vi "OpenAVIFile.vi"(8 "error in (no error)":errorcluster, 11 "AVI Path":path) -> (0 "error out":errorcluster, 3 "Avi Refnum":T1)   [LabVIEW 2016]
uses:
  <vilib>/vision/Avi1.llb/AviRefnum.ctl
  <vilib>/regexp/Match Regular Expression.xnode
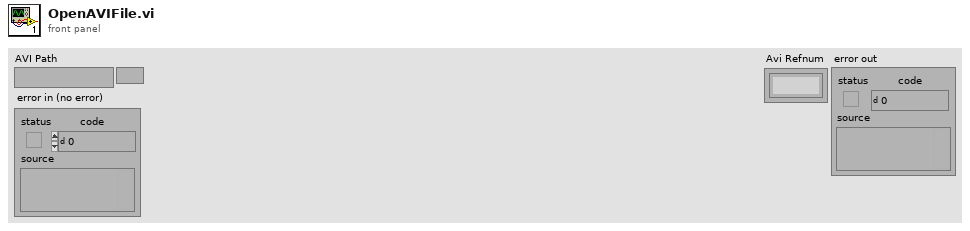
[diagram p1: front panel]
types:
  T1 = typedef "AviRefnum.ctl" = refnum<k1>
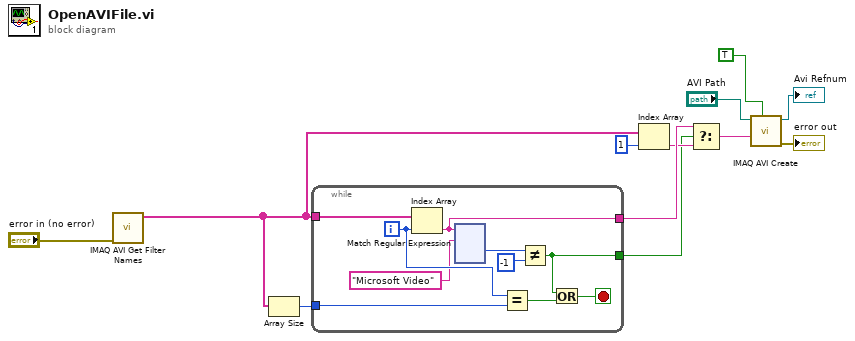
[diagram p0: block diagram]
diagram:
  n1 = call "IMAQ AVI Get Filter Names"("error in (no error)"="error in (no error)") -> ("Filter Names"=w9:string[])  [unwired: 9 in, 1 out]
  n2 = Array Size(array=w9) -> (size(s)=w12:i32)
  n3 = while {
    tunnel: w9 -> [w19]
    tunnel: w12 -> [w22]
    tunnel: [w17] -> w7
    tunnel: [w13] -> w11
    i -> [w18]
    stop <- w21 stop-if-true
    n4 = Index Array(array=w19, index=w18) -> (element=w13:string)
    n5 = xnode "Match Regular Expression"("input string"=w13, "regular expression"="Microsoft Video") -> ("offset past match"=w15:i32)  [unwired: 4 in, 4 out]
    n6 = Equal?(x=w18, y=w22) -> (x = y?=w20:bool)
    n7 = Not Equal?(x=w15, y=-1) -> (x != y?=w17:bool)
    n8 = Or(x=w17, y=w20) -> (x .or. y?=w21:bool)
  }
  n9 = Index Array(array=w9, index=1) -> (element=w8:string)
  n10 = Select(t=w11, s=w7, f=w8) -> (s? t:f=w6:string)
  n11 = call "IMAQ AVI Create"("Has Data"=TRUE, "Compression Filter"=w6, "AVI Path"="AVI Path") -> ("error out"=→"error out":errorcluster, "Avi Refnum"=→"Avi Refnum":T1)  [unwired: 4 in, 3 out]
